vi "NicmosGetFrequencyRange.vi"(2 "Bank Number":i32, 9 "error in (no error)":errorcluster caption="entrée d'erreur") -> (1 "Max Frame Rate":dbl[unit] format="%.2f", 5 "Min Frame Rate":dbl[unit] format="%.2f", 6 "error out":errorcluster caption="sortie d'erreur")   [LabVIEW 2009]
uses:
  NicmosGlobal.vi
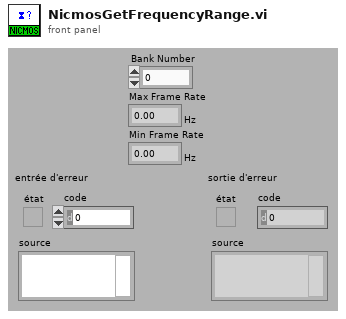
[diagram p1: front panel]
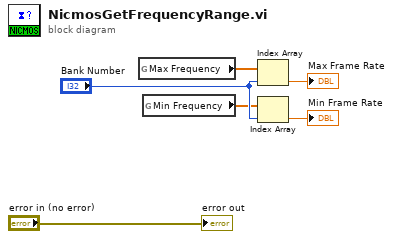
[diagram p0: block diagram]
diagram:
  n1 = global read "NicmosGlobal.vi" "Max Frequency"() -> (w5:dbl[unit][])
  n2 = global read "NicmosGlobal.vi" "Min Frequency"() -> (w4:dbl[unit][])
  n3 = Index Array(array=w5, index="Bank Number") -> (element=→"Max Frame Rate":dbl[unit])
  n4 = Index Array(array=w4, index="Bank Number") -> (element=→"Min Frame Rate":dbl[unit])
  "error out" <- "error in (no error)"
